vi "VNA-FMR_in-plane.vi"() -> ()   [LabVIEW 2015]
panel:
  in  "Shitty Gaussmeter?":bool
  in  "Field Points":i32=150
  out "Current Set Point":dbl
  out "Current Output":dbl
  in  "Global Finished Email":bool
  in  "Save Directory":path=path "C:/Users/probe_station/Desktop/VNA-FMR_Data"
  in  "Scan Email":bool
  in  "Send File":bool
  out "Frequency":string
  out "Sweep Number":dbl
  out "Average IMAG":cluster{dbl[], dbl[]}(graph)
  out "Average REAL":cluster{dbl[], dbl[]}(graph)
  in  "Field Sweeps":i32=5
  out "Sweep IMAG":cluster{dbl[], dbl[]}(graph)
  out "Sweep REAL":cluster{dbl[], dbl[]}(graph)
  out "VNA IMAG":dbl
  out "Field":dbl
  out "VNA REAL":dbl
  in  "Response Cal":bool=TRUE
  in  "Port Power Level":string="0"
  in  "Marker Sweep/Time Point":string="3ms"
  in  "VNA CW Sweep Time":string="min"
  in  "VNA number of Points":string="2"
  in  "Power Supply Address":string="6"
  in  "Current Start (A)":dbl
  in  "Current Stop (A)":dbl=20.0
  in  "VNA Address":string="15"
  in  "GaussMeter Address":string="22"
  in  "Start (GHz)":dbl=8.0
  in  "Stop (GHz)":dbl=9.0
  in  "Frequency Points":i32=2
  in  "Recipient's Email Address Address":string
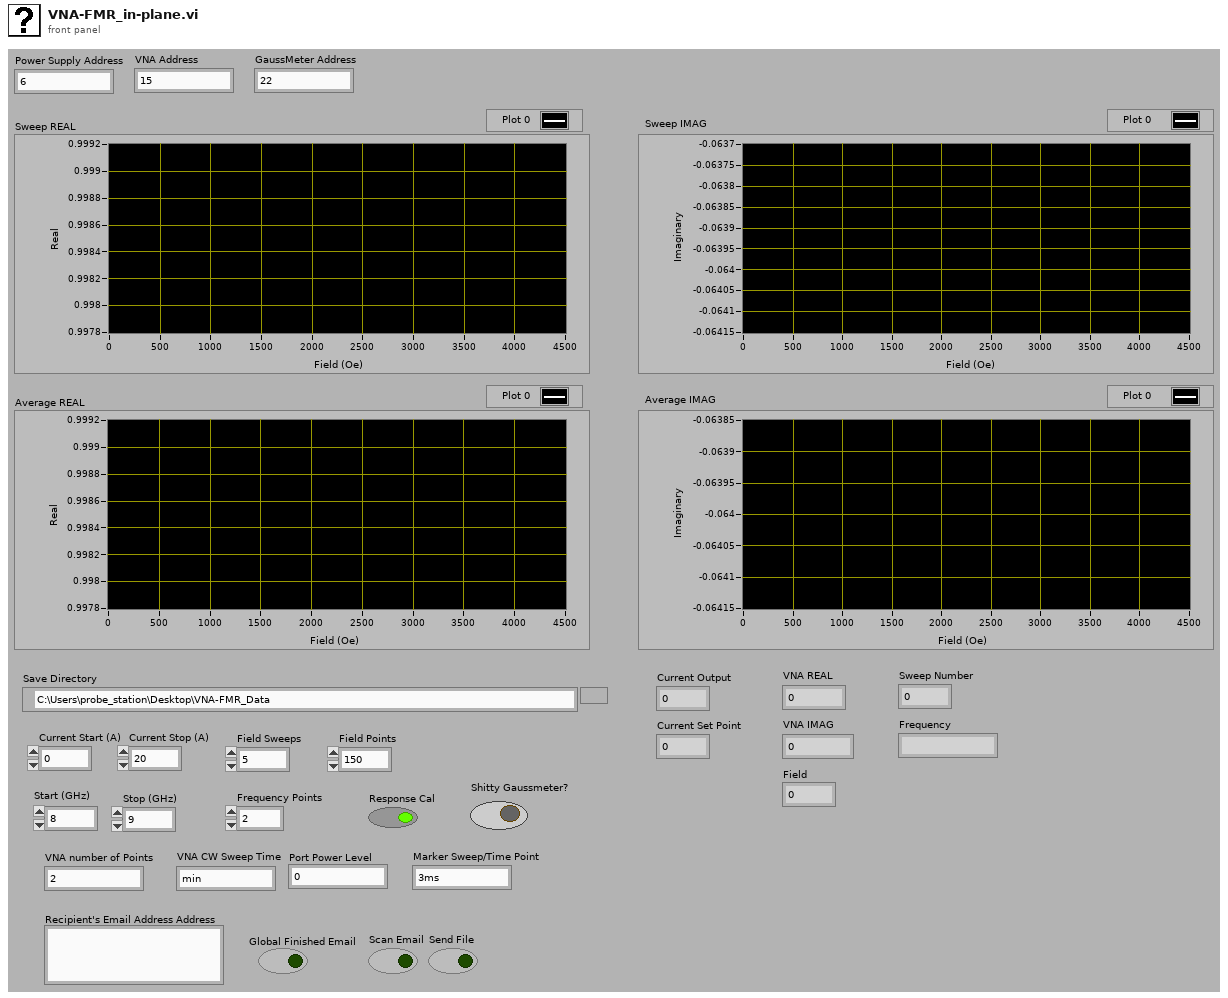
[diagram p1: front panel]
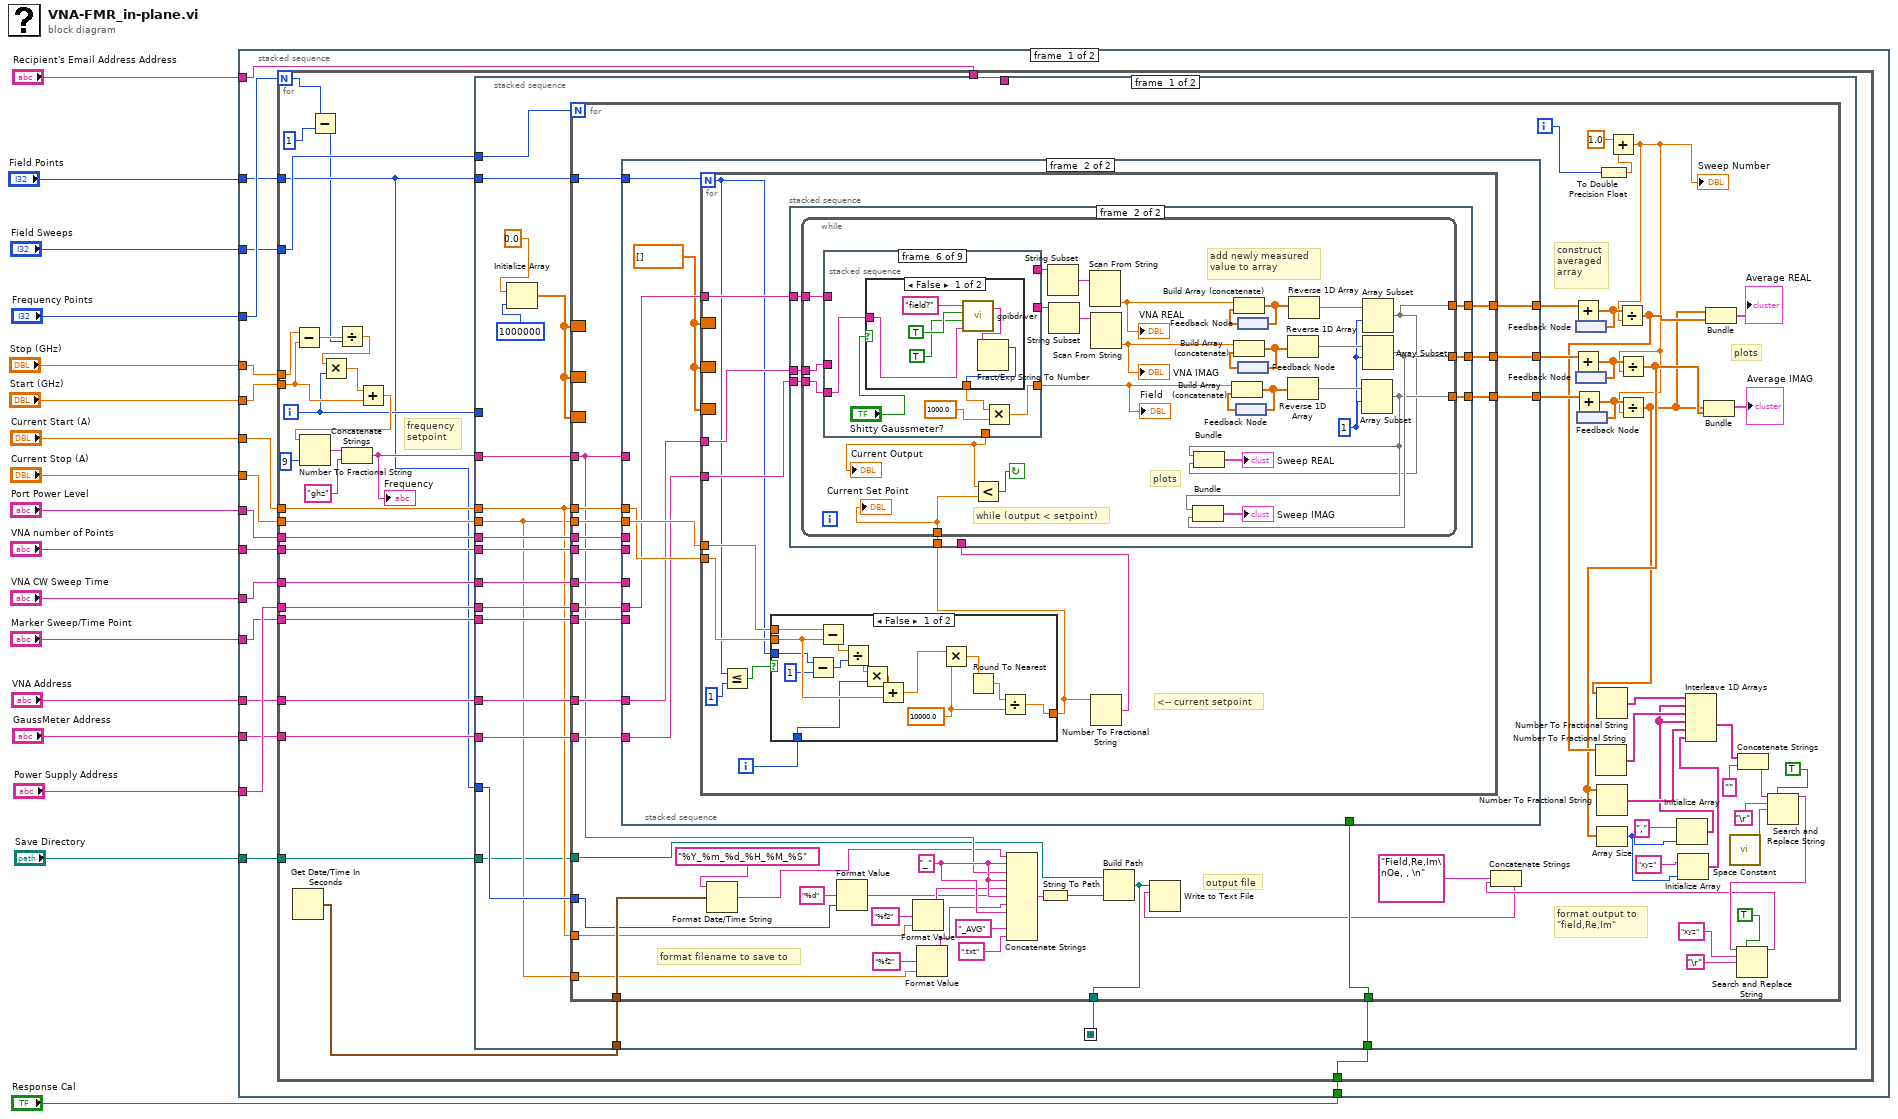
[diagram p0: block diagram]
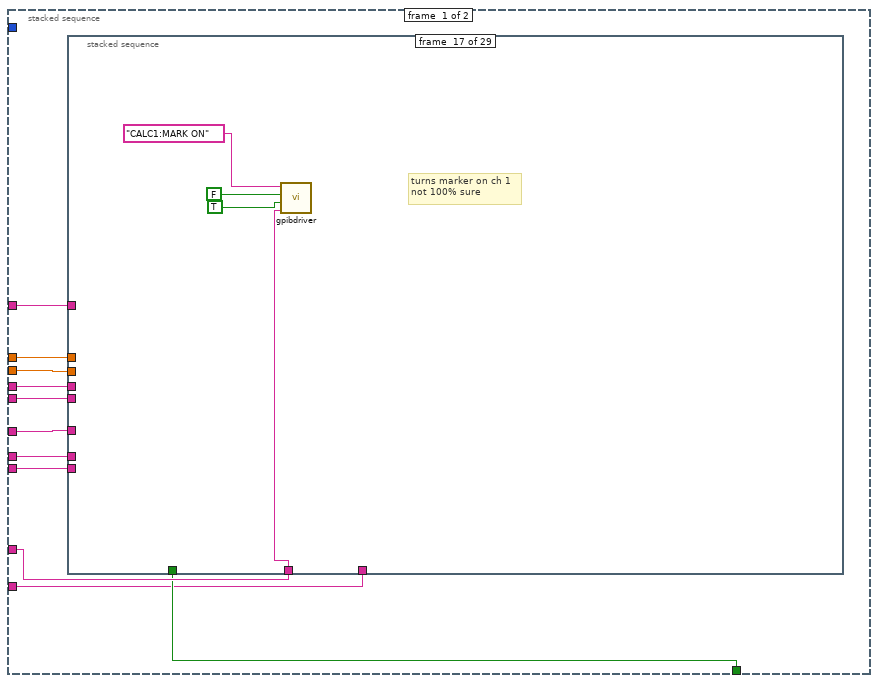
[diagram p2: hidden frame]
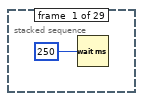
[diagram p3: hidden frame]
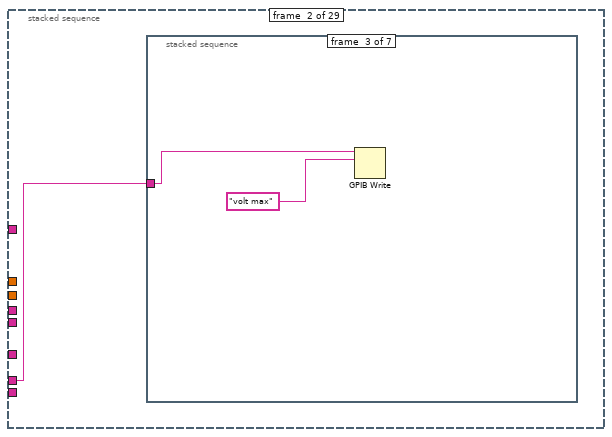
[diagram p4: hidden frame]
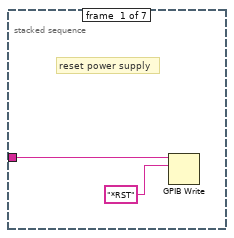
[diagram p5: hidden frame]
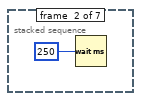
[diagram p6: hidden frame]
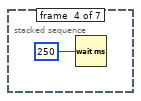
[diagram p7: hidden frame]
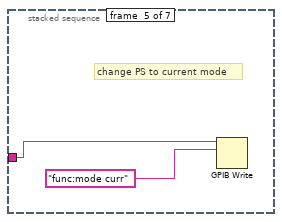
[diagram p8: hidden frame]
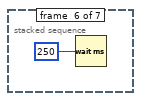
[diagram p9: hidden frame]
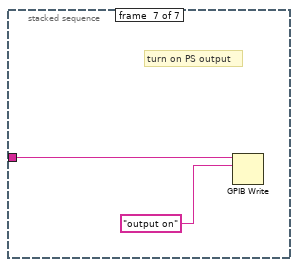
[diagram p10: hidden frame]
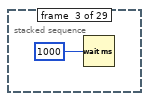
[diagram p11: hidden frame]
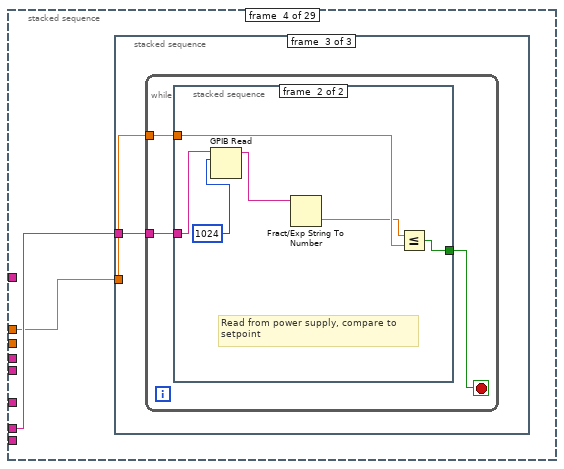
[diagram p12: hidden frame]
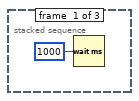
[diagram p13: hidden frame]
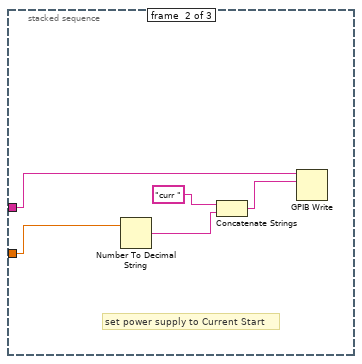
[diagram p14: hidden frame]
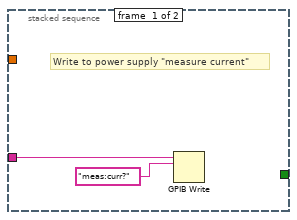
[diagram p15: hidden frame]
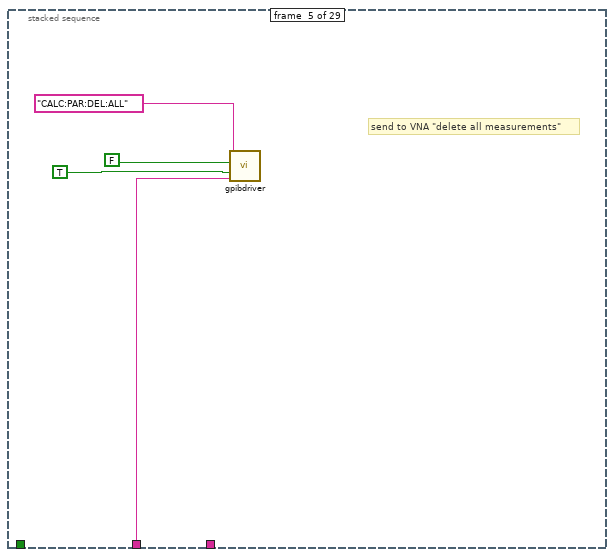
[diagram p16: hidden frame]
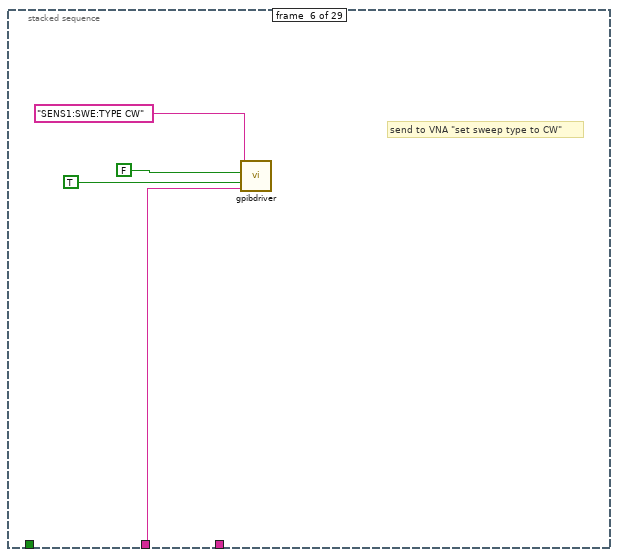
[diagram p17: hidden frame]
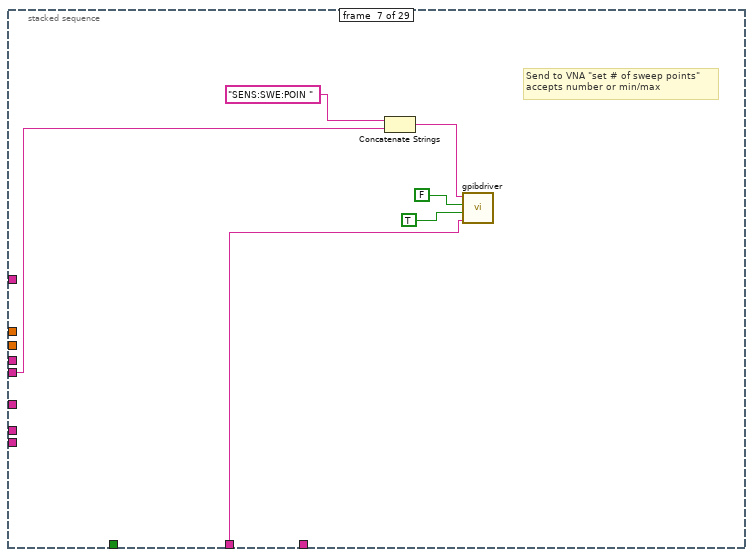
[diagram p18: hidden frame]
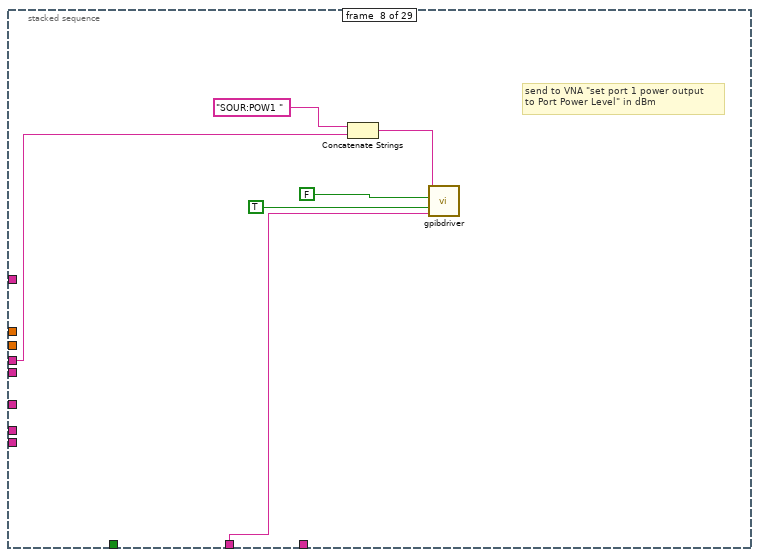
[diagram p19: hidden frame]
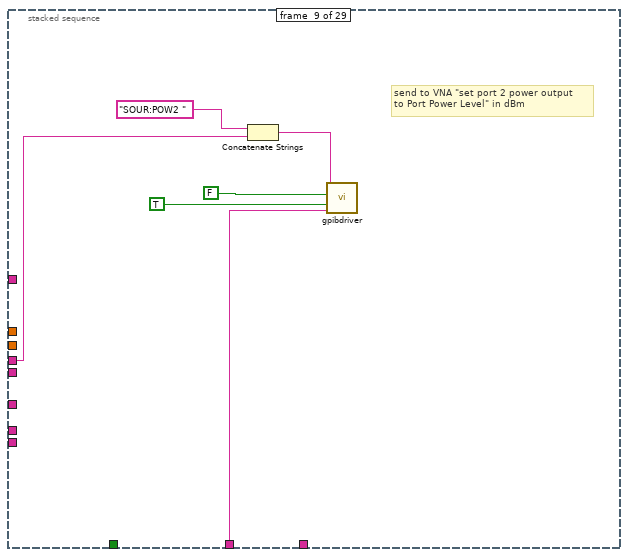
[diagram p20: hidden frame]
diagram:
  n1 = stacked-sequence {
    tunnel: "Recipient's Email Address Address" -> [w19 w496]
    tunnel: "Frequency Points" -> [w34 _]
    tunnel: "Stop (GHz)" -> [w33 _]
    tunnel: "Start (GHz)" -> [w32 _]
    tunnel: "Current Start (A)" -> [w30 _]
    tunnel: "Current Stop (A)" -> [w29 _]
    tunnel: "Port Power Level" -> [w26 _]
    tunnel: "VNA number of Points" -> [w27 _]
    tunnel: "VNA CW Sweep Time" -> [w25 _]
    tunnel: "Marker Sweep/Time Point" -> [w23 _]
    tunnel: "VNA Address" -> [w28 _]
    tunnel: "Power Supply Address" -> [w31 w494]
    tunnel: "GaussMeter Address" -> [w22 _]
    tunnel: "Response Cal" -> [w24 _]
    tunnel: "Field Points" -> [w21 _]
    tunnel: "Field Sweeps" -> [w20 _]
    tunnel: "Save Directory" -> [w18 _]
    frame #0 {
      n2 = for {
        N: w34 -> [w37]
        tunnel: w33 -> [w63]
        tunnel: w32 -> [w59]
        tunnel: w31 -> [w54]
        tunnel: w30 -> [w53]
        tunnel: w29 -> [w52]
        tunnel: w28 -> [w51]
        tunnel: w27 -> [w50]
        tunnel: w26 -> [w49]
        tunnel: w25 -> [w48]
        tunnel: w24 -> [w47]
        tunnel: w23 -> [w46]
        tunnel: w22 -> [w45]
        tunnel: w21 -> [w39]
        tunnel: w20 -> [w44]
        tunnel: w19 -> [w42]
        tunnel: w18 -> [w38]
        i -> [w41]
        # "frequency\nsetpoint"
        n3 = Get Date/Time In Seconds() -> (seconds since 1Jan1904=w40:timestamp)
        n4 = Subtract(x=w63, y=w59) -> (x-y=w62:dbl)
        n5 = Subtract(x=w37, y=1) -> (x-y=w35:i32)
        n6 = Divide(x=w62, y=w35) -> (x/y=w61:dbl)
        n7 = Multiply(x=w61, y=w41) -> (x*y=w60:dbl)
        n8 = Add(x=w60, y=w59) -> (x+y=w55:dbl)
        n9 = Number To Fractional String(number=w55, precision (6)=i16 9) -> (F-format string=w58:string)  [unwired: 2 in]
        n10 = Concatenate Strings(w58, "ghz" ("string")) -> (w43:string)
        "Frequency" <- w43
        n11 = stacked-sequence {
          seq-local: [w64 _] -> [_ w473]
          tunnel: w54 -> [w83 _]
          tunnel: w53 -> [w67 _]
          tunnel: w52 -> [w66 _]
          tunnel: w51 -> [w82 _]
          tunnel: w50 -> [w81 _]
          tunnel: w49 -> [w80 _]
          tunnel: w43 -> [w79 w476]
          tunnel: w48 -> [w78 _]
          tunnel: w47 -> [w77 _]
          tunnel: w46 -> [w76 _]
          tunnel: w45 -> [w75 _]
          tunnel: w39 -> [w74 _]
          tunnel: w44 -> [w73 _]
          tunnel: w42 -> [_ w475]
          tunnel: w41 -> [_ w474]
          tunnel: w40 -> [w69 _]
          tunnel: w39 -> [w68 _]
          tunnel: w38 -> [w65 _]
          frame #0 {
            n12 = Initialize Array(0.0 ("element"), 1000000 ("dimension size")) -> (w70:dbl[])
            n13 = for {
              N: w73 -> [_]
              tunnel: w83 -> [w153]
              tunnel: w67 -> [w152]
              tunnel: w66 -> [w151]
              tunnel: w82 -> [w150]
              tunnel: w81 -> [w149]
              tunnel: w80 -> [w148]
              tunnel: w79 -> [w118]
              tunnel: w78 -> [w147]
              tunnel: w77 -> [w146]
              tunnel: w76 -> [w145]
              tunnel: w75 -> [w144]
              tunnel: w74 -> [w143]
              border: w70 -> [_]
              border: w70 -> [_]
              border: w70 -> [_]
              tunnel: w69 -> [w130]
              tunnel: w68 -> [w128]
              tunnel: w67 -> [w120]
              tunnel: w66 -> [w119]
              tunnel: w65 -> [w116]
              tunnel: [w95] -> w64
              i -> [w85]
              w127 = "_" ("string")
              # "output file"
              # "format filename to save to"
              # "format output to\n\"field,Re,Im\""
              # "construct\naveraged\narray"
              # "plots"
              n14 = stacked-sequence {
                tunnel: w153 -> [w164 w344]
                tunnel: w152 -> [w163 w345]
                tunnel: w151 -> [w162 w346]
                tunnel: w150 -> [w161 w342]
                tunnel: w149 -> [w160 _]
                tunnel: w148 -> [w159 _]
                tunnel: w118 -> [w158 _]
                tunnel: w147 -> [w157 _]
                tunnel: w146 -> [w156 _]
                tunnel: w145 -> [w155 _]
                tunnel: w144 -> [w154 w343]
                tunnel: w143 -> [_ w337]
                tunnel: [_ w340] -> w139
                tunnel: [_ w339] -> w138
                tunnel: [_ w338] -> w137
                frame #0 {
                  n15 = stacked-sequence {
                    tunnel: w164 -> [_ w166 _ w180 _ _ _ _ _ _ _ _ _ _ _ _ _ _ _ _ _ _ _ _ _ _ _ _ w335]
                    tunnel: w163 -> [_ _ _ w179 _ _ _ _ _ _ _ _ _ _ _ _ _ _ _ _ _ _ _ _ _ _ _ _ w334]
                    tunnel: w162 -> [_ _ _ _ _ _ _ _ _ _ _ _ _ _ _ _ _ _ _ _ _ _ _ _ _ _ _ _ w333]
                    tunnel: w161 -> [_ _ _ _ w200 w204 w208 w214 w220 w226 w232 w238 w242 w246 w250 w255 w269 w273 w279 w283 w287 w292 w306 w310 w314 w321 _ _ _]
                    tunnel: w160 -> [_ _ _ _ _ _ w209 _ _ _ _ _ _ _ _ _ _ _ _ _ _ _ _ _ _ _ _ _ _]
                    tunnel: w159 -> [_ _ _ _ _ _ _ w215 w221 _ _ _ _ _ _ _ _ _ _ _ _ _ _ _ _ _ _ _ _]
                    tunnel: w158 -> [_ _ _ _ _ _ _ _ _ w227 _ _ _ _ _ _ _ _ _ _ _ _ _ _ _ _ _ _ _]
                    tunnel: w157 -> [_ _ _ _ _ _ _ _ _ _ w233 _ _ _ _ _ _ _ _ _ _ _ _ _ _ _ _ _ _]
                    tunnel: w156 -> [_ _ _ _ _ _ _ _ _ _ _ _ _ _ _ w254 _ _ _ _ _ w291 _ _ _ _ _ _ _]
                    tunnel: w155 -> [_ _ _ _ _ _ _ _ _ _ _ _ _ _ _ _ _ w274 _ _ _ _ _ _ w315 _ _ _ _]
                    tunnel: w154 -> [_ _ _ _ _ _ _ _ _ _ _ _ _ _ _ _ _ _ _ _ _ _ _ _ _ w320 w328 _ _]
                    frame #0 {
                      n16 = Wait (ms)(milliseconds to wait=u32 250) -> ()  [unwired: 1 out]
                    }
                    frame #1 {
                      n17 = stacked-sequence {
                        tunnel: w166 -> [w167 _ w171 _ w174 _ w177]
                        frame #0 {
                          # "reset power supply"
                          n18 = GPIB Write(0:w167, 1:"*RST" ("data")) -> ()  [unwired: 3 in, 2 out]
                        }
                        frame #1 {
                          n19 = Wait (ms)(milliseconds to wait=u32 250) -> ()  [unwired: 1 out]
                        }
                        frame #2 {
                          n20 = GPIB Write(0:w171, 1:"volt max" ("data")) -> ()  [unwired: 3 in, 2 out]
                        }
                        frame #3 {
                          n21 = Wait (ms)(milliseconds to wait=u32 250) -> ()  [unwired: 1 out]
                        }
                        frame #4 {
                          # "change PS to current mode"
                          n22 = GPIB Write(0:w174, 1:"func:mode curr" ("data")) -> ()  [unwired: 3 in, 2 out]
                        }
                        frame #5 {
                          n23 = Wait (ms)(milliseconds to wait=u32 250) -> ()  [unwired: 1 out]
                        }
                        frame #6 {
                          # "turn on PS output"
                          n24 = GPIB Write(0:w177, 1:"output on" ("data")) -> ()  [unwired: 3 in, 2 out]
                        }
                      }
                    }
                    frame #2 {
                      n25 = Wait (ms)(milliseconds to wait=u32 1000) -> ()  [unwired: 1 out]
                    }
                    frame #3 {
                      n26 = stacked-sequence {
                        tunnel: w180 -> [_ w186 w188]
                        tunnel: w179 -> [_ w183 w187]
                        frame #0 {
                          n27 = Wait (ms)(milliseconds to wait=u32 1000) -> ()  [unwired: 1 out]
                        }
                        frame #1 {
                          # "set power supply to Current Start"
                          n28 = Number To Decimal String(number=w183) -> (decimal integer string=w182:string)  [unwired: 1 in]
                          n29 = Concatenate Strings("curr " ("string"), w182) -> (w184:string)
                          n30 = GPIB Write(0:w186, 1:w184) -> ()  [unwired: 3 in, 2 out]
                        }
                        frame #2 {
                          n31 = while {
                            tunnel: w188 -> [w190]
                            tunnel: w187 -> [w189]
                            stop <- w191 stop-if-true
                            n32 = stacked-sequence {
                              tunnel: [_ w199] -> w191
                              tunnel: w190 -> [w193 w197]
                              tunnel: w189 -> [_ w198]
                              frame #0 {
                                # "Write to power supply \"measure current\""
                                n33 = GPIB Write(0:w193, 1:"meas:curr?" ("data")) -> ()  [unwired: 3 in, 2 out]
                              }
                              frame #1 {
                                # "Read from power supply, compare to\nsetpoint"
                                n34 = GPIB Read(0:w197, 1:1024 ("byte count")) -> (5:w196:string)  [unwired: 3 in, 2 out]
                                n35 = Fract/Exp String To Number(string=w196) -> (number=w195:dbl)  [unwired: 3 in, 1 out]
                                n36 = Less Or Equal?(x=w195, y=w198) -> (x <= y?=w199:bool)
                              }
                            }
                          }
                        }
                      }
                    }
                    frame #4 {
                      # "send to VNA \"delete all measurements\""
                      n37 = call "gpibdriver.vi"("Characters to Write"="CALC:PAR:DEL:ALL", "Read"=FALSE, "Write"=TRUE ("Write 3"), "GPIB\nAddress"=w200) -> ()  [unwired: 2 in, 1 out]
                    }
                    frame #5 {
                      # "send to VNA \"set sweep type to CW\""
                      n38 = call "gpibdriver.vi"("Characters to Write"="SENS1:SWE:TYPE CW", "Read"=FALSE, "Write"=TRUE ("Write 3"), "GPIB\nAddress"=w204) -> ()  [unwired: 2 in, 1 out]
                    }
                    frame #6 {
                      # "Send to VNA \"set # of sweep points\"\naccepts number or min/max"
                      n39 = Concatenate Strings("SENS:SWE:POIN " ("Characters to Write"), w209) -> (w210:string)
                      n40 = call "gpibdriver.vi"("Characters to Write"=w210, "Read"=FALSE, "Write"=TRUE, "GPIB\nAddress"=w208) -> ()  [unwired: 2 in, 1 out]
                    }
                    frame #7 {
                      # "send to VNA \"set port 1 power output\nto Port Power Level\" in dBm"
                      n41 = Concatenate Strings("SOUR:POW1 " ("Characters to Write"), w215) -> (w216:string)
                      n42 = call "gpibdriver.vi"("Characters to Write"=w216, "Read"=FALSE, "Write"=TRUE ("Write 3"), "GPIB\nAddress"=w214) -> ()  [unwired: 2 in, 1 out]
                    }
                    frame #8 {
                      # "send to VNA \"set port 2 power output\nto Port Power Level\" in dBm"
                      n43 = Concatenate Strings("SOUR:POW2 " ("Characters to Write"), w221) -> (w222:string)
                      n44 = call "gpibdriver.vi"("Characters to Write"=w222, "Read"=FALSE, "Write"=TRUE ("Write 3"), "GPIB\nAddress"=w220) -> ()  [unwired: 2 in, 1 out]
                    }
                    frame #9 {
                      # "set VNA frequency to calculated frequency"
                      n45 = Concatenate Strings("SENS:FREQ:CW " ("Characters to Write"), w227) -> (w229:string)
                      n46 = call "gpibdriver.vi"("Characters to Write"=w229, "Read"=FALSE, "Write"=TRUE ("Write 3"), "GPIB\nAddress"=w226) -> ()  [unwired: 2 in, 1 out]
                    }
                    frame #10 {
                      # "set sweep time"
                      n47 = Concatenate Strings("SENS:SWE:TIME " ("Characters to Write"), w233) -> (w234:string)
                      n48 = call "gpibdriver.vi"("Characters to Write"=w234, "Read"=FALSE, "Write"=TRUE ("Write 3"), "GPIB\nAddress"=w232) -> ()  [unwired: 2 in, 1 out]
                    }
                    frame #11 {
                      # "create new VNA measurement of S21"
                      n49 = call "gpibdriver.vi"("Characters to Write"="CALC1:PAR:DEF \"CH1_S21_RE\", S21", "Read"=FALSE, "Write"=TRUE ("Write 3"), "GPIB\nAddress"=w238) -> ()  [unwired: 2 in, 1 out]
                    }
                    frame #12 {
                      # "Display real S21 measurement on VNA"
                      n50 = call "gpibdriver.vi"("Characters to Write"="DISP:WIND1:TRAC1:FEED \"CH1_S21_RE\"", "Read"=FALSE, "Write"=TRUE ("Write 3"), "GPIB\nAddress"=w242) -> ()  [unwired: 2 in, 1 out]
                    }
                    frame #13 {
                      # "sets S21 measurement on VNA"
                      n51 = call "gpibdriver.vi"("Characters to Write"="CALC1:PAR:SEL \"CH1_S21_RE\"", "Read"=FALSE, "Write"=TRUE ("Write 3"), "GPIB\nAddress"=w246) -> ()  [unwired: 2 in, 1 out]
                    }
                    frame #14 {
                      # "display Real part of selected measurement (S21)"
                      n52 = call "gpibdriver.vi"("Characters to Write"="CALC1:FORM REAL", "Read"=FALSE, "Write"=TRUE ("Write 3"), "GPIB\nAddress"=w250) -> ()  [unwired: 2 in, 1 out]
                    }
                    frame #15 {
                      # "Response Cal?"
                      n53 = case shown="True" w254 {
                        tunnel: w255 -> [_ w256]
                        frame False {
                        }
                        frame True {
                          n54 = stacked-sequence {
                            tunnel: w256 -> [w257 w261 w265]
                            frame #0 {
                              # "set ch 1 calibratoin to Response Thru"
                              n55 = call "gpibdriver.vi"("Characters to Write"="SENS:CORR:COLL:METH TRAN1", "Read"=FALSE, "Write"=TRUE, "GPIB\nAddress"=w257) -> ()  [unwired: 2 in, 1 out]
                            }
                            frame #1 {
                              # "measure the calibration standard\n(not 100% sure on this one)"
                              n56 = call "gpibdriver.vi"("Characters to Write"="SENS:CORR:COLL STAN4", "Read"=FALSE, "Write"=TRUE, "GPIB\nAddress"=w261) -> ()  [unwired: 2 in, 1 out]
                            }
                            frame #2 {
                              # "save calibration"
                              n57 = call "gpibdriver.vi"("Characters to Write"="SENS:CORR:COLL:SAVE", "Read"=FALSE, "Write"=TRUE, "GPIB\nAddress"=w265) -> ()  [unwired: 2 in, 1 out]
                            }
                          }
                        }
                      }
                    }
                    frame #16 {
                      # "turns marker on ch 1\nnot 100% sure"
                      n58 = call "gpibdriver.vi"("Characters to Write"="CALC1:MARK ON", "Read"=FALSE, "Write"=TRUE ("Write 3"), "GPIB\nAddress"=w269) -> ()  [unwired: 2 in, 1 out]
                    }
                    frame #17 {
                      # "set ch1 marker to Marker Sweep/Time point"
                      n59 = Concatenate Strings("CALC1:MARK:X " ("Characters to Write"), w274) -> (w275:string)
                      n60 = call "gpibdriver.vi"("Characters to Write"=w275, "Read"=FALSE, "Write"=TRUE ("Write 3"), "GPIB\nAddress"=w273) -> ()  [unwired: 2 in, 1 out]
                    }
                    frame #18 {
                      # "create new S21 measurement"
                      n61 = call "gpibdriver.vi"("Characters to Write"="CALC1:PAR:DEF \"CH1_S21_IM\", S21", "Read"=FALSE, "Write"=TRUE ("Write 3"), "GPIB\nAddress"=w279) -> ()  [unwired: 2 in, 1 out]
                    }
                    frame #19 {
                      # "display imaginary S21 measurement\non VNA"
                      n62 = call "gpibdriver.vi"("Characters to Write"="DISP:WIND1:TRAC2:FEED \"CH1_S21_IM\"", "Read"=FALSE, "Write"=TRUE ("Write 3"), "GPIB\nAddress"=w283) -> ()  [unwired: 2 in, 1 out]
                    }
                    frame #20 {
                      # "select Im S21 measurement"
                      n63 = call "gpibdriver.vi"("Characters to Write"="CALC1:PAR:SEL \"CH1_S21_IM\"", "Read"=FALSE, "Write"=TRUE ("Write 3"), "GPIB\nAddress"=w287) -> ()  [unwired: 2 in, 1 out]
                    }
                    frame #21 {
                      # "response cal?"
                      n64 = case shown="True" w291 {
                        tunnel: w292 -> [_ w293]
                        frame False {
                        }
                        frame True {
                          n65 = stacked-sequence {
                            tunnel: w293 -> [w294 w298 w302]
                            frame #0 {
                              # "set calibratoin to response thru"
                              n66 = call "gpibdriver.vi"("Characters to Write"="SENS:CORR:COLL:METH TRAN1", "Read"=FALSE, "Write"=TRUE, "GPIB\nAddress"=w294) -> ()  [unwired: 2 in, 1 out]
                            }
                            frame #1 {
                              # "measure calibration?"
                              n67 = call "gpibdriver.vi"("Characters to Write"="SENS:CORR:COLL STAN4", "Read"=FALSE, "Write"=TRUE, "GPIB\nAddress"=w298) -> ()  [unwired: 2 in, 1 out]
                            }
                            frame #2 {
                              # "save calibration"
                              n68 = call "gpibdriver.vi"("Characters to Write"="SENS:CORR:COLL:SAVE", "Read"=FALSE, "Write"=TRUE, "GPIB\nAddress"=w302) -> ()  [unwired: 2 in, 1 out]
                            }
                          }
                        }
                      }
                    }
                    frame #22 {
                      n69 = call "gpibdriver.vi"("Characters to Write"="CALC1:FORM IMAG", "Read"=FALSE, "Write"=TRUE ("Write 3"), "GPIB\nAddress"=w306) -> ()  [unwired: 2 in, 1 out]
                    }
                    frame #23 {
                      n70 = call "gpibdriver.vi"("Characters to Write"="CALC1:MARK ON", "Read"=FALSE, "Write"=TRUE ("Write 3"), "GPIB\nAddress"=w310) -> ()  [unwired: 2 in, 1 out]
                    }
                    frame #24 {
                      n71 = Concatenate Strings("CALC1:MARK:X " ("Characters to Write"), w315) -> (w316:string)
                      n72 = call "gpibdriver.vi"("Characters to Write"=w316, "Read"=FALSE, "Write"=TRUE ("Write 3"), "GPIB\nAddress"=w314) -> ()  [unwired: 2 in, 1 out]
                    }
                    frame #25 {
                      # "set fast data mode on gauss meter\nshould this be outside this structure/\nhigher level?"
                      # "set manual sweep on VNA"
                      n73 = call "gpibdriver.vi"("Characters to Write"="INIT:CONT OFF", "Read"=FALSE, "Write"=TRUE, "GPIB\nAddress"=w321) -> ()  [unwired: 2 in, 1 out]
                      n74 = call "gpibdriver.vi"("Characters to Write"="fast 1", "Read"=FALSE, "Write"=TRUE, "GPIB\nAddress"=w320) -> ()  [unwired: 2 in, 1 out]
                    }
                    frame #26 {
                      # "set highest range on gauss meter"
                      n75 = call "gpibdriver.vi"("Characters to Write"="range 0", "Read"=FALSE, "Write"=TRUE ("Write 3"), "GPIB\nAddress"=w328) -> ()  [unwired: 2 in, 1 out]
                    }
                    frame #27 {
                      n76 = Wait (ms)(milliseconds to wait=u32 250) -> ()  [unwired: 1 out]
                    }
                    frame #28 {
                      # "Why is there another structure nested\nin here?"
                      n77 = stacked-sequence {
                        tunnel: w335 -> [_ _ _ _]
                        tunnel: w334 -> [_ _ _ _]
                        tunnel: w333 -> [_ _ _ _]
                        frame #0 {
                          # "turn on PS\n-> removed"
                        }
                        frame #1 {
                          n78 = Wait (ms)(milliseconds to wait=u32 50) -> ()  [unwired: 1 out]
                        }
                        frame #2 {
                          # "->removed\n\ncurrent from PS > current start?"
                        }
                        frame #3 {
                          # "set PS to Current Stop\n-> removed\n\nI don't think I need to do this"
                        }
                      }
                    }
                  }
                }
                frame #1 {
                  w341 = dbl[] []
                  n79 = for {
                    N: w337 -> [w350]
                    tunnel: w346 -> [w352]
                    tunnel: w345 -> [w353]
                    tunnel: w344 -> [w360]
                    tunnel: w343 -> [w359]
                    tunnel: w342 -> [w358]
                    border: w341 -> [_]
                    border: w341 -> [_]
                    border: w341 -> [_]
                    tunnel: [w357] -> w340
                    tunnel: [w356] -> w339
                    tunnel: [w355] -> w338
                    i -> [w351]
                    # "<-- current setpoint"
                    n80 = Less Or Equal?(x=w350, y=1) -> (x <= y?=w354:bool)
                    n81 = case shown="False" w354 {
                      tunnel: w350 -> [w365 _]
                      tunnel: w353 -> [w370 w379]
                      tunnel: w352 -> [w369 w378]
                      tunnel: w351 -> [w368 _]
                      tunnel: [w361 w375] -> w348
                      frame False {
                        w362 = 10000.0 ("y")
                        n82 = Subtract(x=w365, y=1) -> (x-y=w366:i32)
                        n83 = Subtract(x=w369, y=w370) -> (x-y=w374:dbl)
                        n84 = Divide(x=w374, y=w366) -> (x/y=w372:dbl)
                        n85 = Multiply(x=w372, y=w368) -> (x*y=w371:dbl)
                        n86 = Add(x=w371, y=w370) -> (x+y=w373:dbl)
                        n87 = Multiply(x=w373, y=w362) -> (x*y=w364:dbl)
                        n88 = Round To Nearest(number=w364) -> (nearest integer value=w363:dbl)
                        n89 = Divide(x=w363, y=w362) -> (x/y=w361:dbl)
                      }
                      frame True {
                        n90 = Subtract(x=w378, y=w379) -> (x-y=w381:dbl)
                        n91 = Divide(x=w381, y=1.0) -> (x/y=w377:dbl)
                        n92 = Add(x=w377, y=w379) -> (x+y=w380:dbl)
                        n93 = Multiply(x=w380, y=1.0) -> (x*y=w375:dbl)
                      }
                    }
                    n94 = Number To Fractional String(number=w348) -> (F-format string=w347:string)  [unwired: 3 in]
                    n95 = stacked-sequence {
                      tunnel: w360 -> [w383 w388]
                      tunnel: w347 -> [w385 _]
                      tunnel: w359 -> [_ w393]
                      tunnel: w358 -> [_ w392]
                      tunnel: [_ w391] -> w357
                      tunnel: [_ w390] -> w356
                      tunnel: [_ w389] -> w355
                      tunnel: w348 -> [_ w387]
                      frame #0 {
                        n96 = Concatenate Strings("curr " ("string"), w385) -> (w384:string)
                        n97 = GPIB Write(0:w383, 1:w384) -> ()  [unwired: 3 in, 2 out]
                      }
                      frame #1 {
                        n98 = while {
                          tunnel: w393 -> [w421]
                          tunnel: w392 -> [w420]
                          tunnel: [w399] -> w391
                          tunnel: [w401] -> w390
                          tunnel: [w400] -> w389
                          tunnel: w388 -> [w398]
                          tunnel: w387 -> [w396]
                          stop <- w397 continue-if-true
                          w404 = 1 ("index")
                          # "add newly measured\nvalue to array"
                          # "while (output < setpoint)"
                          # "plots"
                          n99 = stacked-sequence {
                            tunnel: w421 -> [_ _ _ _ _ w448 _ _ _]
                            tunnel: w420 -> [w422 w426 w431 w435 w440 _ w457 _ _]
                            tunnel: [_ _ w430 _ _ _ _ _ _] -> w419
                            tunnel: [_ _ _ _ w439 _ _ _ _] -> w418
                            tunnel: w398 -> [_ _ _ _ _ _ _ w461 w472]
                            tunnel: [_ _ _ _ _ _ _ _ w463] -> w395
                            tunnel: [_ _ _ _ _ w445 _ _ _] -> w394
                            frame #0 {
                              # "send trigger to VNA"
                              n100 = call "gpibdriver.vi"("Characters to Write"="INIT", "Read"=FALSE, "Write"=TRUE ("Write 2"), "GPIB\nAddress"=w422) -> ()  [unwired: 2 in, 1 out]
                            }
                            frame #1 {
                              # "select Re S21 measurement"
                              n101 = call "gpibdriver.vi"("Characters to Write"="CALC1:PAR:SEL \"CH1_S21_RE\"", "Read"=FALSE, "Write"=TRUE ("Write 2"), "GPIB\nAddress"=w426) -> ()  [unwired: 2 in, 1 out]
                            }
                            frame #2 {
                              # "read Re S21 value, output"
                              n102 = call "gpibdriver.vi"("Characters to Write"="CALC1:MARK:Y? ", "Read"=TRUE, "Write"=TRUE ("Write 3"), "GPIB\nAddress"=w431) -> ("Characters Read"=w430:string)  [unwired: 2 in]
                            }
                            frame #3 {
                              # "select Im S21 measurement"
                              n103 = call "gpibdriver.vi"("Characters to Write"="CALC1:PAR:SEL \"CH1_S21_IM\"", "Read"=FALSE, "Write"=TRUE ("Write 3"), "GPIB\nAddress"=w435) -> ()  [unwired: 2 in, 1 out]
                            }
                            frame #4 {
                              # "read Im S21 value, output"
                              n104 = call "gpibdriver.vi"("Characters to Write"="CALC1:MARK:Y? ", "Read"=TRUE, "Write"=TRUE ("Write 3"), "GPIB\nAddress"=w440) -> ("Characters Read"=w439:string)  [unwired: 2 in]
                            }
                            frame #5 {
                              n105 = case shown="False" "Shitty Gaussmeter?" {
                                tunnel: w448 -> [w451 w456]
                                tunnel: [w449 w455] -> w444
                                frame False {
                                n106 = call "gpibdriver.vi"("Characters to Write"="field?", "Read"=TRUE, "Write"=TRUE ("Write 2"), "GPIB\nAddress"=w451) -> ("Characters Read"=w450:string)  [unwired: 2 in]
                                n107 = Fract/Exp String To Number(string=w450) -> (offset past number=w449:i32)  [unwired: 3 in, 1 out]
                                }
                                frame True {
                                # "read field value, output"
                                n108 = call "Field_from_HP3478A.vi"("GPIB Address"=w456) -> ("kOe"=w455:dbl)  [unwired: 2 out]
                                }
                              }
                              n109 = Multiply(x=w444, y=1000.0) -> (x*y=w445:dbl)
                            }
                            frame #6 {
                              # "operation complete?"
                              n110 = call "gpibdriver.vi"("Characters to Write"="*OPC?", "Read"=TRUE, "Write"=TRUE ("Write 2"), "GPIB\nAddress"=w457) -> ()  [unwired: 2 in, 1 out]
                            }
                            frame #7 {
                              # "query current from PS"
                              n111 = GPIB Write(0:w461, 1:"meas:curr?" ("data")) -> ()  [unwired: 3 in, 2 out]
                            }
                            frame #8 {
                              w466 = 1000.0 ("y")
                              # "find Current Output,\ndon't stall, output"
                              n112 = GPIB Read(0:w472, 1:1024 ("byte count")) -> (5:w470:string)  [unwired: 3 in, 2 out]
                              n113 = Fract/Exp String To Number(string=w470) -> (number=w469:dbl)  [unwired: 3 in, 1 out]
                              n114 = Multiply(x=w469, y=w466) -> (x*y=w468:dbl)
                              n115 = Round To Nearest(number=w468) -> (nearest integer value=w467:dbl)
                              n116 = Divide(x=w467, y=w466) -> (x/y=w465:dbl)
                              n117 = Add(x=w465, y=0.005) -> (x+y=w463:dbl)
                            }
                          }
                          "Field" <- w394
                          "Current Output" <- w395
                          n118 = Less?(x=w395, y=w396) -> (x < y?=w397:bool)
                          n119 = String Subset(string=w419) -> (substring=w417:string)  [unwired: 2 in]
                          n120 = String Subset(string=w418) -> (substring=w416:string)  [unwired: 2 in]
                          n121 = Scan From String(input string=w417) -> (output 1=w411:dbl)  [unwired: 4 in, 3 out]
                          "VNA REAL" <- w411
                          n122 = Scan From String(input string=w416) -> (output 1=w412:dbl)  [unwired: 4 in, 3 out]
                          "VNA IMAG" <- w412
                          n123 = feedback #1() -> (w415:dbl[])
                          n124 = Build Array (concatenate)(w394, w415) -> (w408:dbl[])
                          n125 = feedback-in #1(w408) -> ()
                          n126 = feedback #2() -> (w413:dbl[])
                          n127 = Build Array (concatenate)(w411, w413) -> (w409:dbl[])
                          n128 = feedback-in #2(w409) -> ()
                          n129 = feedback #3() -> (w414:dbl[])
                          n130 = Build Array (concatenate)(w412, w414) -> (w410:dbl[])
                          n131 = feedback-in #3(w410) -> ()
                          n132 = Reverse 1D Array(array=w410) -> (reversed array=w406:dbl[])
                          n133 = Reverse 1D Array(array=w408) -> (reversed array=w405:dbl[])
                          n134 = Reverse 1D Array(array=w409) -> (reversed array=w407:dbl[])
                          n135 = Array Subset(array=w405, index=w404) -> (w400:dbl[])  [unwired: 1 in]
                          n136 = Array Subset(array=w407, index=w404) -> (w399:dbl[])  [unwired: 1 in]
                          n137 = Bundle(w400, w399) -> (→"Sweep REAL":cluster{dbl[], dbl[]})  [unwired: 1 in]
                          n138 = Array Subset(array=w406, index=w404) -> (w401:dbl[])  [unwired: 1 in]
                          n139 = Bundle(w400, w401) -> (→"Sweep IMAG":cluster{dbl[], dbl[]})  [unwired: 1 in]
                          "Current Set Point" <- w396
                        }
                      }
                    }
                  }
                }
              }
              n140 = Format Date/Time String(time format string (%c)="%Y_%m_%d_%H_%M_%S", seconds (now)=w130) -> (date/time string=w93:string)  [unwired: 1 in]
              n141 = Format Value(format string="%d", value (0)=w128) -> (output string=w94:string)  [unwired: 1 in]
              n142 = Format Value(format string="%f2", value (0)=w120) -> (output string=w125:string)  [unwired: 1 in]
              n143 = Format Value(format string="%f2", value (0)=w119) -> (output string=w126:string)  [unwired: 1 in]
              n144 = Concatenate Strings(w93, w127, w118, w127, w125, w127, w126, w127, w94, "_AVG" ("string"), ".txt" ("string")) -> (w117:string)
              n145 = String To Path(string=w117) -> (path=w115:path)
              n146 = Build Path(base path=w116, name or relative path=w115) -> (appended path=w95:path)
              n147 = feedback #4() -> (w142:dbl[])
              n148 = Add(x=w139, y=w142) -> (x+y=w136:dbl[])
              n149 = feedback-in #4(w136) -> ()
              n150 = feedback #5() -> (w141:dbl[])
              n151 = Add(x=w138, y=w141) -> (x+y=w135:dbl[])
              n152 = feedback-in #5(w135) -> ()
              n153 = feedback #6() -> (w140:dbl[])
              n154 = Add(x=w137, y=w140) -> (x+y=w134:dbl[])
              n155 = feedback-in #6(w134) -> ()
              n156 = To Double Precision Float(number=w85) -> (double precision float=w87:dbl)
              n157 = Add(x=1.0, y=w87) -> (x+y=w84:dbl)
              "Sweep Number" <- w84
              n158 = Divide(x=w136, y=w84) -> (x/y=w114:dbl[])
              n159 = Number To Fractional String(number=w114) -> (F-format string=w98:string[])  [unwired: 3 in]
              n160 = Divide(x=w135, y=w84) -> (x/y=w113:dbl[])
              n161 = Number To Fractional String(number=w113) -> (F-format string=w97:string[])  [unwired: 3 in]
              n162 = Array Size(array=w113) -> (size(s)=w96:i32)
              n163 = Divide(x=w134, y=w84) -> (x/y=w92:dbl[])
              n164 = Number To Fractional String(number=w92) -> (F-format string=w99:string[])  [unwired: 3 in]
              n165 = Initialize Array(",", w96) -> (w91:string[])
              n166 = Initialize Array("xyz" ("element"), w96) -> (w101:string[])
              n167 = Interleave 1D Arrays(w99, w91, w98, w91, w97, w101) -> (w103:string[])
              n168 = Bundle(w92, w113) -> (→"Average IMAG":cluster{dbl[], dbl[]})  [unwired: 1 in]
              n169 = Bundle(w92, w114) -> (→"Average REAL":cluster{dbl[], dbl[]})  [unwired: 1 in]
              n170 = call <vilib>:"Space Constant.vi"() -> ("String"=w112:string)
              n171 = Concatenate Strings(w103, "" ("string")) -> (w104:string)
              n172 = Search and Replace String(replace all?=TRUE ("replace all? (F)"), input string=w104, search string="\r", replace string=w112) -> (result string=w106:string)  [unwired: 4 in, 3 out]
              n173 = Search and Replace String(replace all?=TRUE ("replace all? (F)"), input string=w106, search string="xyz", replace string="\r") -> (result string=w89:string)  [unwired: 4 in, 3 out]
              n174 = Concatenate Strings("Field,Re,Im\nOe, , \n" ("string"), w89) -> (w88:string)
              n175 = Write to Text File(file (use dialog)=w95, text=w88) -> ()  [unwired: 2 in, 3 out]
            }
          }
          frame #1 {
            n176 = case shown="True" "Scan Email" {
              tunnel: w476 -> [_ w481]
              tunnel: w475 -> [_ w480]
              tunnel: w474 -> [_ w479]
              tunnel: w473 -> [_ w478]
              frame False {
              }
              frame True {
                n177 = case shown="True" "Send File" {
                  tunnel: w481 -> [w486 w492]
                  tunnel: w480 -> [w484 w489]
                  tunnel: w479 -> [_ _]
                  tunnel: w478 -> [_ w488]
                  frame False {
                    n178 = Concatenate Strings("Scan Finished @ " ("Body"), w486) -> (w483:string)
                    n179 = call "gmail 8.2.vi"("Subject"="VNA-FMR System Message", "Body"=w483, "Recipient's Email Address Address"=w484) -> ()  [unwired: 8 in, 1 out]
                  }
                  frame True {
                    n180 = Concatenate Strings("Scan Finished @ " ("Body"), w492) -> (w490:string)
                    n181 = call "gmail 8.2.vi"("Attachment - Optional"=w488, "Subject"="VNA-FMR System Message", "Body"=w490, "Recipient's Email Address Address"=w489) -> ()  [unwired: 7 in, 1 out]
                  }
                }
              }
            }
          }
        }
      }
    }
    frame #1 {
      n182 = case shown="True" "Global Finished Email" {
        tunnel: w496 -> [_ w500]
        frame False {
        }
        frame True {
          n183 = call "gmail 8.2.vi"("Subject"="VNA-FMR System Message", "Body"="All Points Finished", "Recipient's Email Address Address"=w500) -> ()  [unwired: 8 in, 1 out]
        }
      }
      n184 = GPIB Write(0:w494, 1:"*RST;syst:beep" ("data")) -> ()  [unwired: 3 in, 2 out]
    }
  }
